vi "attributes-owner-test.vi"(8 "error in (no error)":errorcluster) -> (0 "error out":errorcluster)   [LabVIEW 2013]
uses:
  src/Support/Attribute.Owner/Attribute.Owner.lvclass/Attribute.Owner.ctl
  src/Support/Attribute/Attribute.lvclass/Attribute.ctl
  <vilib>/Utility/LVClass/Get LV Class Name.vi
  <vilib>/addons/_JKI Toolkits/Caraya/classes/Test/Test.lvclass
  <vilib>/addons/_JKI Toolkits/Caraya/classes/Assert/Assert.lvclass
  src/Support/Attribute/Attribute.lvclass
  src/Support/Attribute.Owner/Attribute.Owner.lvclass
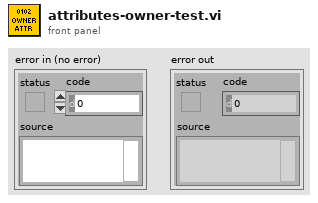
[diagram p1: front panel]
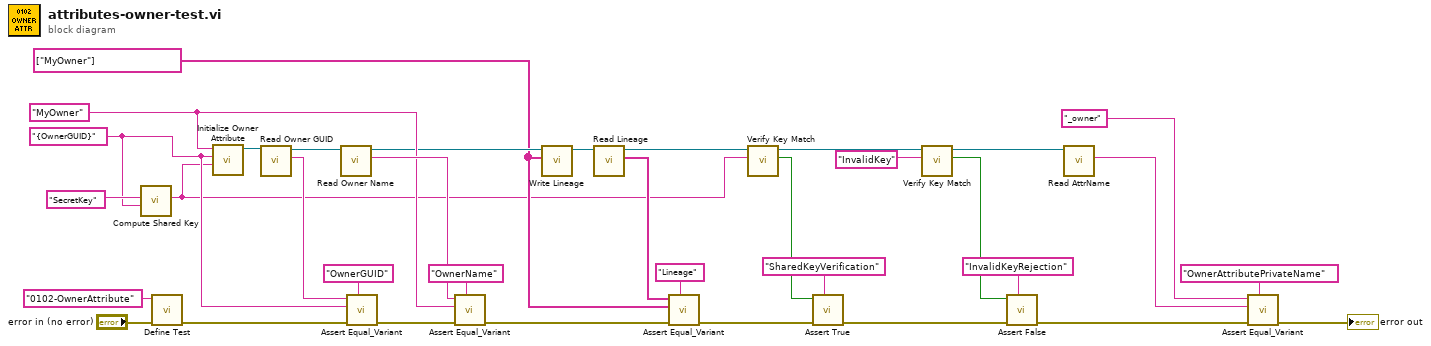
[diagram p0: block diagram]
diagram:
  w16 = string[] ["MyOwner"] ("Lineage")
  w13 = "{OwnerGUID}" ("Name")
  w21 = "MyOwner" ("Name")
  n1 = call "Compute Shared Key.vi"("GUID"=w13, "SecretKey"="SecretKey" ("Name")) -> ("Shared Key"=w11:string)  [unwired: 9 in]
  n2 = call <vilib>:"Define Test.vi"("error in (no error)"="error in (no error)", "Label (VI Title)"="0102-OwnerAttribute") -> ("error out"=w34:errorcluster)  [unwired: 9 in]
  n3 = call "Initialize Owner Attribute.vi"("Shared Key"=w11, "Owner GUID"=w13, "Owner Name"=w21) -> ("Attribute.Owner"=w27:refnum<class "Attribute.Owner.lvclass">)  [unwired: 8 in]
  n4 = call "Read Owner GUID.vi"("Attribute.Owner in"=w27) -> ("Owner GUID"=w26:string, "Attribute.Owner out"=w25:refnum<class "Attribute.Owner.lvclass">)  [unwired: 8 in, 1 out]
  n5 = call "Read Owner Name.vi"("Attribute.Owner in"=w25) -> ("Owner Name"=w22:string, "Attribute.Owner out"=w20:refnum<class "Attribute.Owner.lvclass">)  [unwired: 8 in, 1 out]
  n6 = call <vilib>:"Assert Equal_Variant.vi"("Label"="OwnerGUID" ("Label (VI Title)"), "error in (no error)"=w34, "Y"=w13, "X"=w26) -> ("error out"=w23:errorcluster)  [unwired: 7 in]
  n7 = call <vilib>:"Assert Equal_Variant.vi"("Label"="OwnerName" ("Label (VI Title)"), "error in (no error)"=w23, "Y"=w21, "X"=w22) -> ("error out"=w18:errorcluster)  [unwired: 7 in]
  n8 = call "Write Lineage.vi"("Lineage"=w16, "Attribute.Owner in"=w20) -> ("Attribute.Owner out"=w19:refnum<class "Attribute.Owner.lvclass">)  [unwired: 8 in, 1 out]
  n9 = call "Read Lineage.vi"("Attribute.Owner in"=w19) -> ("Lineage"=w17:string[], "Attribute.Owner out"=w12:refnum<class "Attribute.Owner.lvclass">)  [unwired: 8 in, 1 out]
  n10 = call <vilib>:"Assert Equal_Variant.vi"("Label"="Lineage" ("Label (VI Title)"), "error in (no error)"=w18, "Y"=w16, "X"=w17) -> ("error out"=w9:errorcluster)  [unwired: 7 in]
  n11 = call "Verify Key Match.vi"("Shared Key"=w11, "Attribute.Owner in"=w12) -> ("key matched"=w10:bool, "Attribute.Owner out"=w7:refnum<class "Attribute.Owner.lvclass">)  [unwired: 6 in, 2 out]
  n12 = call <vilib>:"Assert True.vi"("Label"="SharedKeyVerification" ("Label (VI Title)"), "error in (no error)"=w9, "True?"=w10) -> ("error out"=w3:errorcluster)  [unwired: 8 in]
  n13 = call "Verify Key Match.vi"("Shared Key"="InvalidKey" ("Name"), "Attribute.Owner in"=w7) -> ("key matched"=w1:bool, "Attribute.Owner out"=w6:refnum<class "Attribute.Owner.lvclass">)  [unwired: 6 in, 2 out]
  n14 = call <vilib>:"Assert False.vi"("Label"="InvalidKeyRejection" ("Label (VI Title)"), "error in (no error)"=w3, "False?"=w1) -> ("error out"=w2:errorcluster)  [unwired: 8 in]
  n15 = call "Read AttrName.vi"("Attribute in"=w6) -> ("Attribute Name"=w29:string)  [unwired: 9 in, 1 out]
  n16 = call <vilib>:"Assert Equal_Variant.vi"("Label"="OwnerAttributePrivateName" ("Label (VI Title)"), "error in (no error)"=w2, "Y"=w29, "X"="_owner" ("Label (VI Title)")) -> ("error out"=→"error out":errorcluster)  [unwired: 7 in]
